vi "test.vi"() -> ()   [LabVIEW 2014, in "Generic Data Acquisition.lvlib" / "National Instrument USB-6501.lvlib" / "National Instrument USB-6501.lvclass"]
uses:
  National Instrument USB-6501.lvclass
  Controls/Data Acquisition Channel Settings.ctl
  <vilib>/ActorFramework/Message Enqueuer/Message Enqueuer.lvclass/Message Enqueuer.ctl
  National Instrument USB-6501 Messages/Write channel Msg/Write channel Msg.lvclass/Write channel Msg.ctl
  <vilib>/ActorFramework/Message Enqueuer/Enqueue.vi
  <vilib>/ActorFramework/Message Priority Queue/Priority Enqueue.vi
  <vilib>/ActorFramework/Stop Msg/Stop Msg.lvclass
  National Instrument USB-6501 Messages/Write channel Msg/Write channel Msg.lvclass
  SetUp VIs/SetUp VIs.lvlib
  <vilib>/ActorFramework/Actor/Actor.lvclass
panel:
  in  "index of Channel":i32
  in  "Play Button":bool
  in  "Stop Button":bool
  out "Array of line":T1(array[cluster])=[{"Function"=enum."Digital Output", "Port"=0.0, "Line"=0.0}]
  out "error out":errorcluster
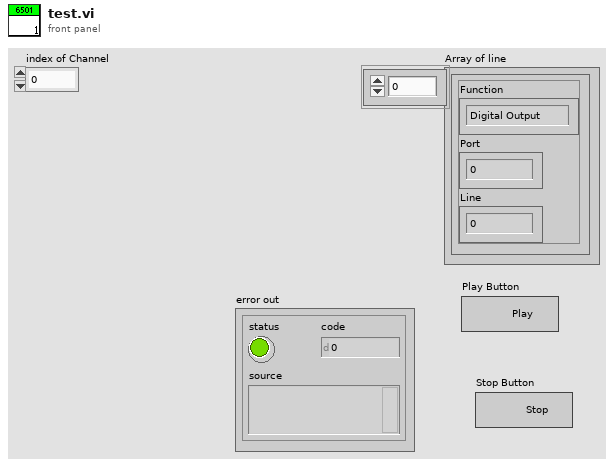
[diagram p1: front panel]
types:
  T1 = cluster{"Function":enum16{"Digital Input", "Digital Output"}, "Port":dbl, "Line":dbl}[]
  T2 = typedef "Data Acquisition Channel Settings.ctl" = cluster{"Function":enum16{"Digital Input", "Digital Output"}, "Port":i8, "Line":i8, "Name":string}
  T3 = cluster{"Manufacturer":string, "Model":string, "Serial":string, "Address":string, "Boolean":bool}[]
  T4 = cluster{"Manufacturer":string, "Model":string, "Serial":string, "Address":string, "Boolean":bool}
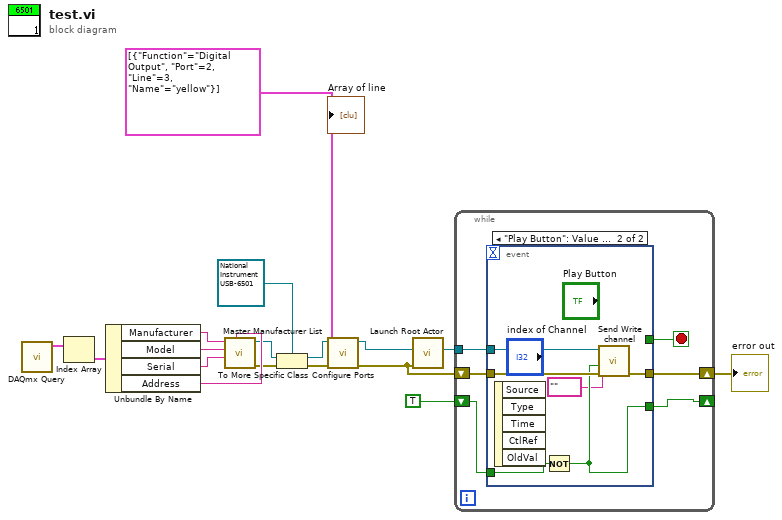
[diagram p0: block diagram]
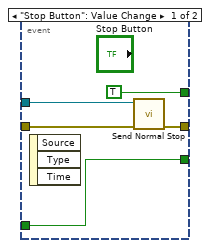
[diagram p2: hidden frame]
diagram:
  n1 = call "DAQmx Query.vi"() -> ("Array"=w17:T3)  [unwired: 3 in, 8 out]
  n2 = Index Array(array=w17) -> (element=w16:T4)  [unwired: 1 in]
  n3 = Unbundle By Name(w16) -> ("Manufacturer"=w15:string, "Model"=w14:string, "Serial"=w13:string, "Address"=w12:string)
  n4 = call "Master Manufacturer List.vi"("VISA resource name"=w12, "Serial"=w13, "Model"=w14, "Manufacturer"=w15) -> ("error out"=w8:errorcluster, "Generic Instrument out"=w11:refnum<class "Generic Instrument.lvclass">)  [unwired: 6 in]
  n5 = To More Specific Class(target class=refnum<class "National Instrument USB-6501.lvclass"> refnum ("Generic Data Acquisition.lvlib:National Instrument USB-6501.lvlib:National Instrument USB-6501.lvclass"), reference=w11, error in=w8) -> (specific class reference=w9:refnum<class "National Instrument USB-6501.lvclass">, error out=w7:errorcluster)
  n6 = call-dynamic "Configure Ports.vi"("error in (no error)"=w7, "Array of line"=T2[] [{"Function"=enum."Digital Output", "Port"=2, "Line"=3, "Name"="yellow"}], "National Instrument USB-6501 in"=w9) -> ("error out"=w3:errorcluster, "National Instrument USB-6501 out"=w4:refnum<class "National Instrument USB-6501.lvclass">)  [unwired: 7 in]
  n7 = call <vilib>:"Launch Root Actor.vi"("error in (no error)"=w3, "Actor"=w4) -> ("Actor's Enqueuer"=w6:refnum<class "Message Enqueuer.lvclass">)  [unwired: 8 in, 1 out]
  n8 = while {
    tunnel: w6 -> [w22]
    shift-right: [w21] -> w5
    shift-left: w3 -> [w20]
    shift-right: [w19] -> _
    shift-left: TRUE ("data") -> [w18]
    stop <- w23 stop-if-true
    n9 = event shown="[1] \"Play Button\": Value Change" {
      selector: _ -> [_ _]
      dyn-events: _ -> [_ _]
      timeout: _ -> [_ _]
      tunnel: [TRUE _] -> w23
      tunnel: w22 -> [w27 w34]
      tunnel: [w26 w33] -> w21
      tunnel: w20 -> [w25 w32]
      tunnel: [w24 w31] -> w19
      tunnel: w18 -> [w24 w30]
      event "Stop Button": Value Change {
        n10 = event-data() -> ()  [unwired: 1 in, 3 out]
        n11 = call <vilib>:"Send Normal Stop.vi"("error in (no error)"=w25, "Message Enqueuer"=w27) -> ("error out"=w26:errorcluster)  [unwired: 9 in]
      }
      event "Play Button": Value Change {
        n12 = event-data() -> ()  [unwired: 1 in, 5 out]
        n13 = Not(x=w30) -> (.not. x?=w31:bool)
        n14 = call "Send Write channel.vi"("error in (no error)"=w32, "data"=w31, "DAQmx Physical Channel"=tag "", "Message Enqueuer"=w34) -> ("error out"=w33:errorcluster)  [unwired: 6 in, 1 out]
      }
    }
  }
  "error out" <- w5
